vi "GetRegisters.vi"(8 "error in (no error)":errorcluster, 9 "Lenght":u8, 10 "Addr":u8[](array[numeric])=[0], 11 "BME680 in":refnum<class "BME680.lvclass">) -> (0 "error out":errorcluster, 2 "Data out":u8[](array[numeric]), 3 "BME680 out":refnum<class "BME680.lvclass">)   [LabVIEW 2022 SP3, in "BME680.lvlib" / "BME680.lvclass"]
uses:
  BME680.lvclass
  BME680.lvclass/BME680.ctl
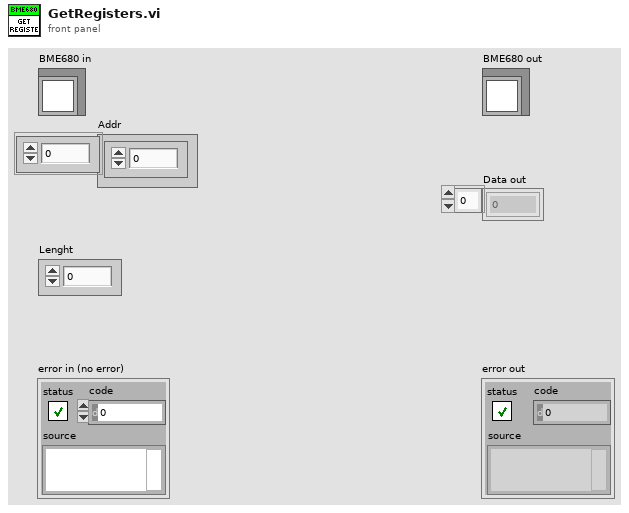
[diagram p1: front panel]
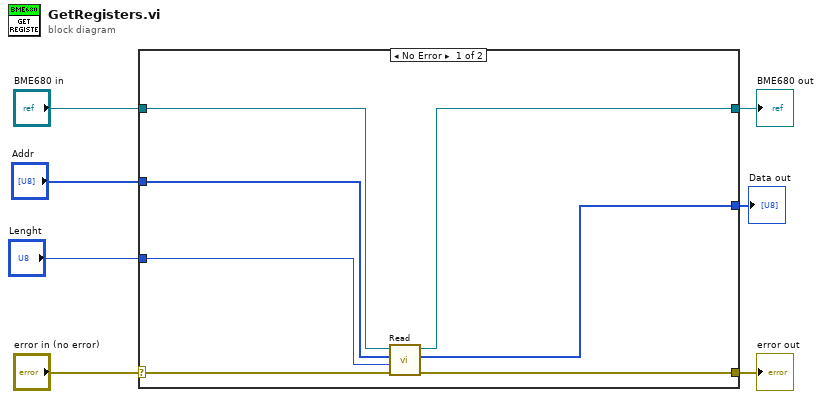
[diagram p0: block diagram]
diagram:
  n1 = case shown="No Error" "error in (no error)" {
    selector: "error in (no error)" -> [w14 w16]
    tunnel: [w13 w16] -> w6
    tunnel: [w9 w15] -> w4
    tunnel: "BME680 in" -> [w12 w15]
    tunnel: "Addr" -> [w11 _]
    tunnel: "Lenght" -> [w10 _]
    tunnel: [w8 _] -> w1
    frame No Error {
      n2 = call "Read.vi"("error in (no error)"=w14, "Bytes To Read"=w10, "Registers"=w11, "BME68x in"=w12) -> ("error out"=w13:errorcluster, "Data out"=w8:u8[], "BME68x out"=w9:refnum<class "BME680.lvclass">)  [unwired: 5 in]
    }
    frame Error {
    }
  }
  "error out" <- w6
  "BME680 out" <- w4
  "Data out" <- w1
